vi "Temperature Measurement.vi"() -> ()   [LabVIEW 2010]
panel:
  out "Average Temp":dbl
  in  "While Loop Delay":dbl(knob) scale=0.0..2.0
  in  "stop":bool
  out "String":string
  in  "Unit":bool
  out "Temperature":dbl
  out "Thermometer":dbl(slide) scale=0.0..100.0
  out "Temp. in C":dbl
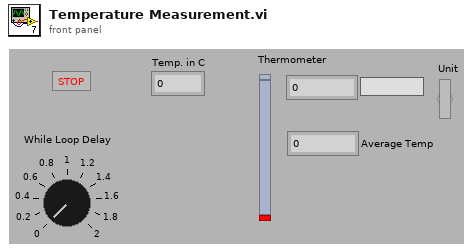
[diagram p1: front panel]
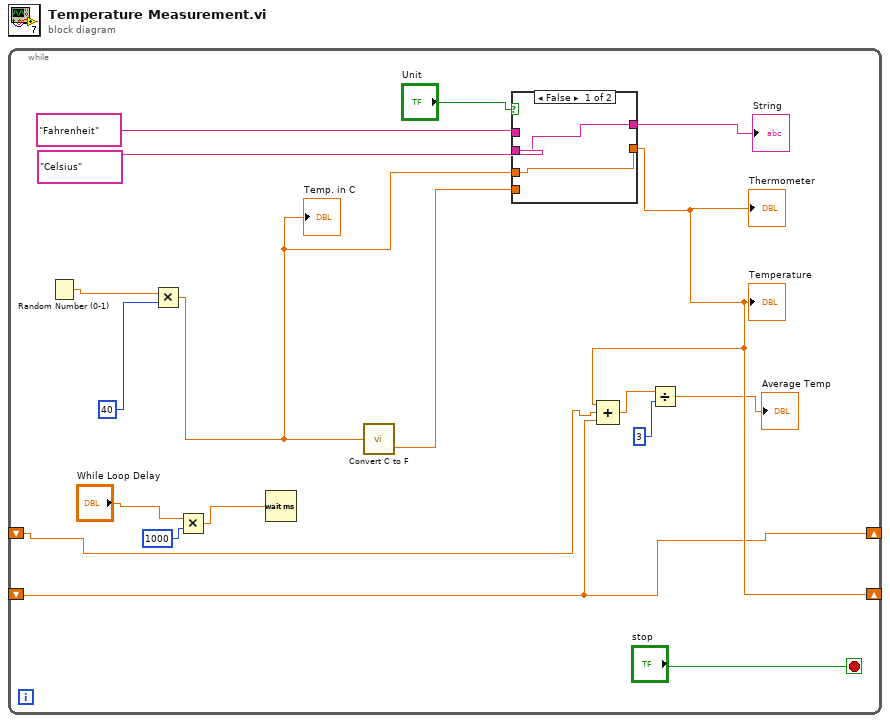
[diagram p0: block diagram]
diagram:
  n1 = while {
    shift-right: [w1] -> _
    shift-left: _ -> [w2]
    shift-right: [w6] -> _
    shift-left: _ -> [w1]
    stop <- "stop" stop-if-true
    n2 = Random Number (0-1)() -> (number: 0 to 1=w18:dbl)
    n3 = Multiply(x=w18, y=40) -> (x*y=w16:dbl)
    "Temp. in C" <- w16
    n4 = Multiply(x="While Loop Delay", y=1000) -> (x*y=w7:dbl)
    n5 = Wait (ms)(milliseconds to wait=w7) -> ()  [unwired: 1 out]
    n6 = call "Convert C to F.vi"("Temp in C"=w16) -> ("Temp in F"=w15:dbl)  [unwired: 1 in]
    n7 = case shown="False" "Unit" {
      tunnel: w16 -> [w20 _]
      tunnel: w15 -> [_ w22]
      tunnel: [w20 w22] -> w6
      tunnel: "Celsius" -> [w19 _]
      tunnel: "Fahrenheit" -> [_ w21]
      tunnel: [w19 w21] -> w11
      frame False {
      }
      frame True {
      }
    }
    "Thermometer" <- w6
    "Temperature" <- w6
    "String" <- w11
    n8 = Compound Arithmetic op=ADD(w6, w2, w1) -> (w4:dbl)
    n9 = Divide(x=w4, y=3) -> (x/y=→"Average Temp":dbl)
  }
